vi "Read Key.vi"(7 "Key:":string, 8 "error in":errorcluster, 11 "Configuration in":refnum<class "Configuration.lvclass">) -> (0 "error out":errorcluster, 2 "Value":string, 3 "Configuration out":refnum<class "Configuration.lvclass">)   [LabVIEW 2018, in "Configuration.lvlib" / "Configuration.lvclass"]
doc: "Read a specific key value from the configuration data."
uses:
  Configuration.lvclass
  Configuration.lvclass/Configuration.ctl
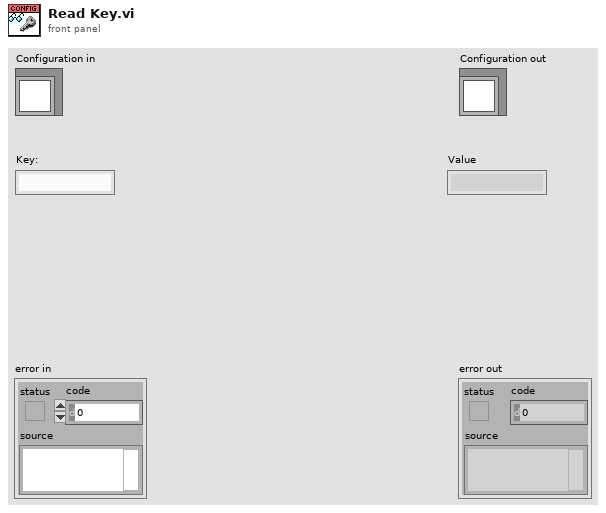
[diagram p1: front panel]
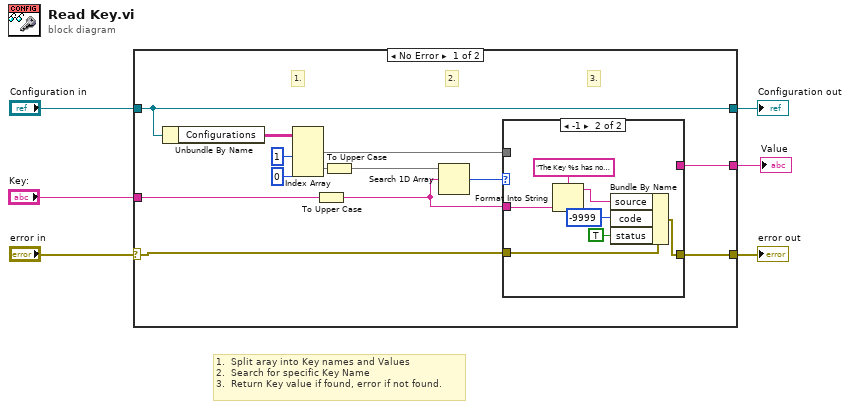
[diagram p0: block diagram]
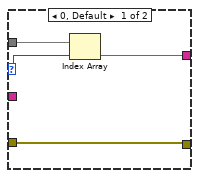
[diagram p2: hidden frame]
diagram:
  # "1.  Split aray into Key names and Values\n2.  Search for specific Key Name\n3.  Return Key value if found, error if not found."
  n1 = case shown="No Error" "error in" {
    selector: "error in" -> [w8 w32]
    tunnel: [w7 w32] -> w5
    tunnel: [w19 w31] -> w3
    tunnel: "Configuration in" -> [w19 w31]
    tunnel: "Key:" -> [w15 _]
    tunnel: [w10 _] -> w1
    frame No Error {
      # "3."
      # "2."
      # "1."
      n2 = Unbundle By Name(w19) -> ("Configurations"=w18:string[][])
      n3 = Index Array(array=w18, index (col) #1=1 ("disabled index (col)"), index (col) #2=0 ("index (col)")) -> (element #1=w13:string[], element #2=w14:string[])  [unwired: 2 in]
      n4 = To Upper Case(1:w15) -> (0:w9:string)
      n5 = To Upper Case(1:w14) -> (0:w12:string[])
      n6 = Search 1D Array(1D array=w12, element=w9) -> (index of element=w11:i32)  [unwired: 1 in]
      n7 = case shown="-1" w11 {
        selector: w11 -> [w22 _]
        tunnel: w13 -> [w23 _]
        tunnel: [w21 _] -> w10
        tunnel: w9 -> [_ w30]
        tunnel: w8 -> [w20 w28]
        tunnel: [w20 w27] -> w7
        frame 0, Default {
          n8 = Index Array(array=w23, index=w22) -> (element=w21:string)
        }
        frame -1 {
          n9 = Format Into String(format string="The Key %s has not been configured", w30) -> (resulting string=w25:string)  [unwired: 2 in, 1 out]
          n10 = Bundle By Name(cluster=w28, "source"=w25, "code"=-9999, "status"=TRUE) -> (w27:errorcluster)
        }
      }
    }
    frame Error {
    }
  }
  "error out" <- w5
  "Configuration out" <- w3
  "Value" <- w1
